vi "Read FTT Subpanel data.vi"(8 "error in (no error)":errorcluster, 11 "Main":T1={"Tite"="", "Base path"=path "", "Table"=[], "Stations"=[], "Shield Array"=[], "UPHs"=[], "VISA"={"VISA"="", "baud rate"=9600, "data bits"=8, "parity"=enum."None", "stop bits"=10, "flow control"=0}, "Path"={"roof"=path "", "Config"=path "", "Png"=path ""}, "Ctr"={"DB Dispaly"=refnum, "Error Table"=refnum, "Display"=refnum, "Login"=refnum, "Exit"=refnum, "FTT_Submit"=refnum}, "Login"={"User"="", "Grade"=""}, "information"={"cause"="", "Type"=enum."Inform", "code"=0, "Suroce"="", "Status"=FALSE}, "Local DB"={"Connstr"="", "Database"={"Constr"={"Driver"="", "Server"="", "User"="", "Pwd"="", "Database"=""}, "conn ref"=refnum, "State"=FALSE}}, "Remote DB"={"Connstr"="", "Database"={"Constr"={"Driver"="", "Server"="", "User"="", "Pwd"="", "Database"=""}, "conn ref"=refnum, "State"=FALSE}}, "FTT TV"="", "ExchangeTime"=0, "NVH"="", "EOL Path"=path ""} {"VISA"."flow control" items=["None", "XON/XOFF", "RTS/CTS", "XON/XOFF & RTS/CTS", "DTR/DSR", "XON/XOFF & DTR/DSR"]; "VISA"."stop bits" items=["1.0"=10, "1.5"=15, "2.0"=20]}) -> (0 "error out":errorcluster)   [LabVIEW 2014]
uses:
  Type'def/FTT Display Type.ctl
  <vilib>/addons/database/_DB Variant To Data/Database Variant To Data.xnode
  Type'def/UPH Config.ctl
  VISA/Ctr/VISA Ctr.ctl
  Type'def/Main Ctr Ref.ctl
  Type'def/User Login.ctl
  Database/Ctr/Constr.ctl
  <vilib>/addons/database/Connection.llb/Conn ObjectReference.ctl
  <vilib>/addons/database/NI_Database_API.lvlib
  Database/Ctr/Conneect State.ctl
  Type'def/MainCtr.ctl
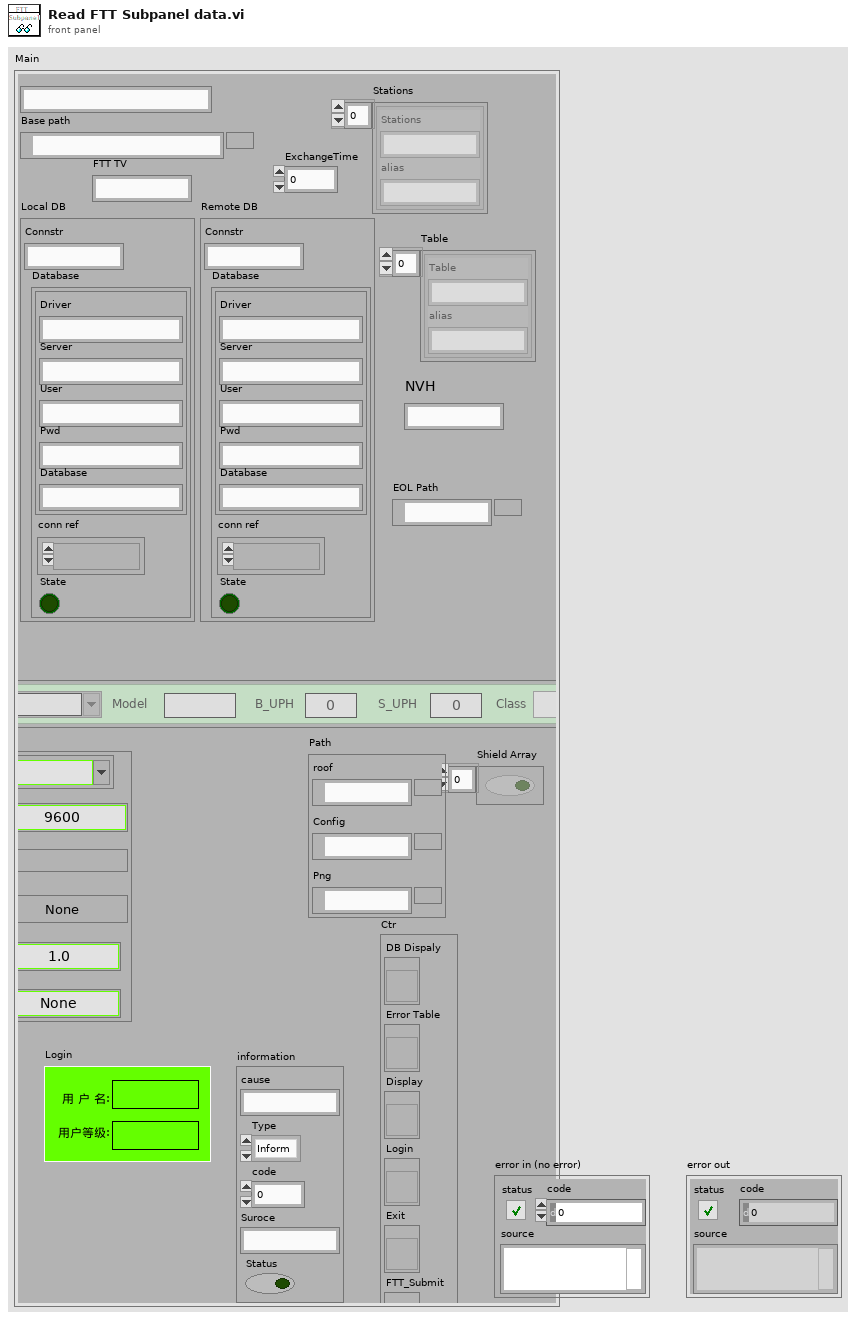
[diagram p1: front panel]
types:
  T1 = typedef "MainCtr.ctl" = cluster{"Tite":string, "Base path":path, "Table":cluster{"Table":string, "alias":string}[], "Stations":cluster{"Stations":string, "alias":string}[], "Shield Array":bool[], "UPHs":T2[], "VISA":T3, "Path":cluster{"roof":path, "Config":path, "Png":path}, "Ctr":T4, "Login":T5, "information":cluster{"cause":string, "Type":enum16{"Inform", "Warning", "Alarm"}, "code":i32, "Suroce":string, "Status":bool}, "Local DB":cluster{"Connstr":string, "Database":T6}, "Remote DB":cluster{"Connstr":string, "Database":T6}, "FTT TV":string, "ExchangeTime":i32, "NVH":string, "EOL Path":path}
  T2 = typedef "UPH Config.ctl" = cluster{"Line_No":string, "Model":string, "B_UPH ":i16, "S_UPH  ":i16, "Class":enum16{"Big", "Small"}}
  T3 = typedef "VISA Ctr.ctl" = cluster{"VISA":refnum<visa-resource-name>, "baud rate":u32, "data bits":u16, "parity":enum16{"None", "Odd", "Even", "Mark", "Space"}, "stop bits":u16, "flow control":u16}
  T4 = typedef "Main Ctr Ref.ctl" = cluster{"DB Dispaly":refnum<vi>, "Error Table":refnum<vi>, "Display":refnum<vi>, "Login":refnum<vi>, "Exit":refnum<vi>, "FTT_Submit":refnum<vi>}
  T5 = typedef "User Login.ctl" = cluster{"User":string, "Grade":string}
  T6 = typedef "Conneect State.ctl" = cluster{"Constr":T7, "conn ref":T8, "State":bool}
  T7 = typedef "Constr.ctl" = cluster{"Driver":string, "Server":string, "User":string, "Pwd":string, "Database":string}
  T8 = typedef "NI_Database_API.lvlib/Conn ObjectReference.ctl" = refnum<k1>
  T9 = typedef "FTT Display Type.ctl" = cluster{"Line.No":string, "Model":string, "Color":string, "UPH":dbl, "Plan":dbl, "Target Rate":dbl, "Target ":dbl, "Actual":dbl, "FTT":dbl, "FTT Rate":dbl, "Repaired":dbl, "Reject":dbl, "Ouline":dbl, "Line State":string}
  T10 = cluster{"cause":string, "Type":enum16{"Inform", "Warning", "Alarm"}, "code":i32, "Suroce":string, "Status":bool}
  T11 = cluster{"Main ":T1, "Display":T9, "information":cluster{"cause":string, "Type":enum16{"Inform", "Warning", "Alarm"}, "code":i32, "Suroce":string, "Status":bool}}
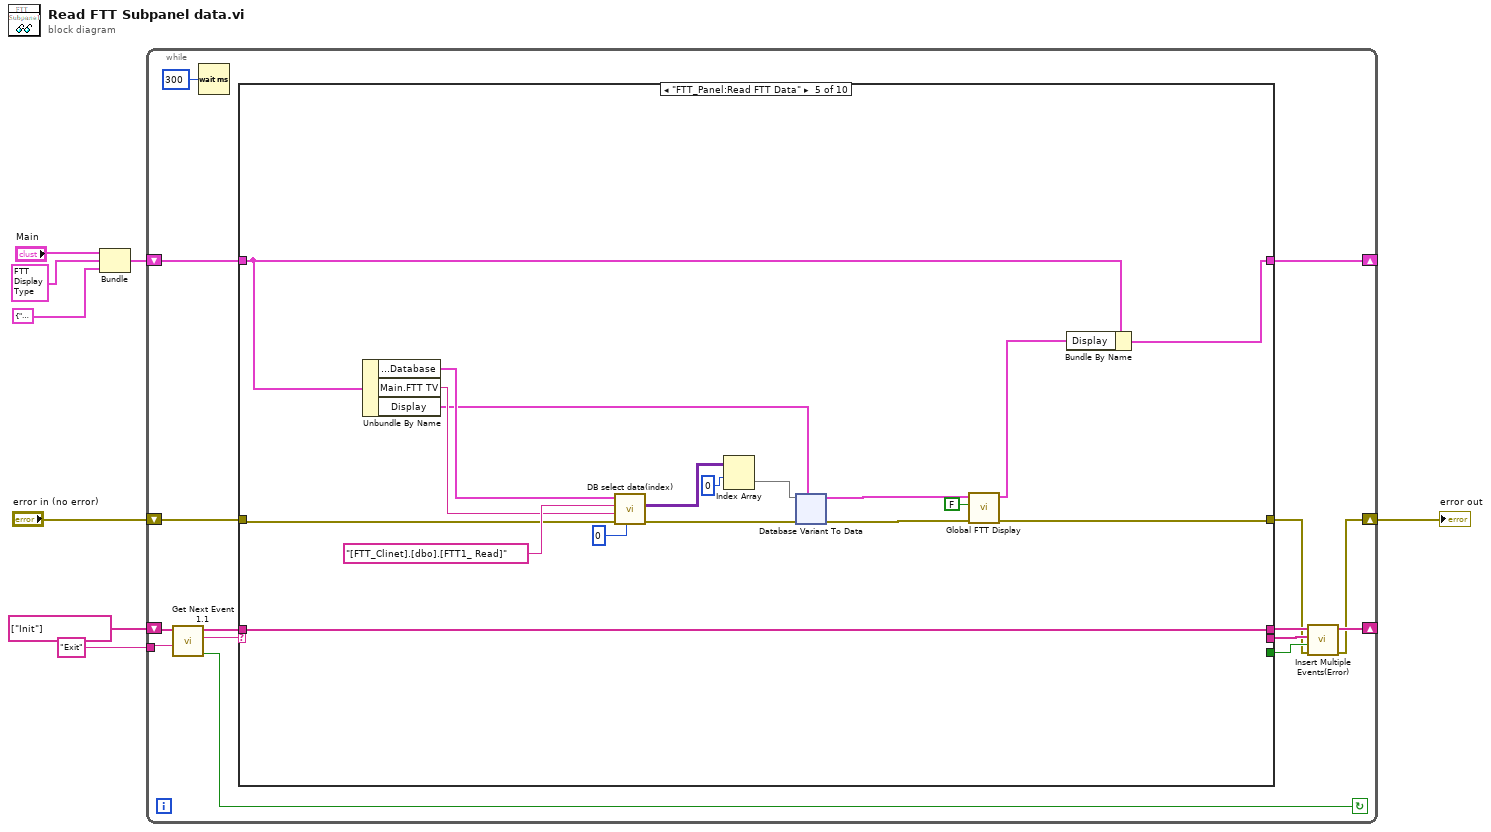
[diagram p0: block diagram]
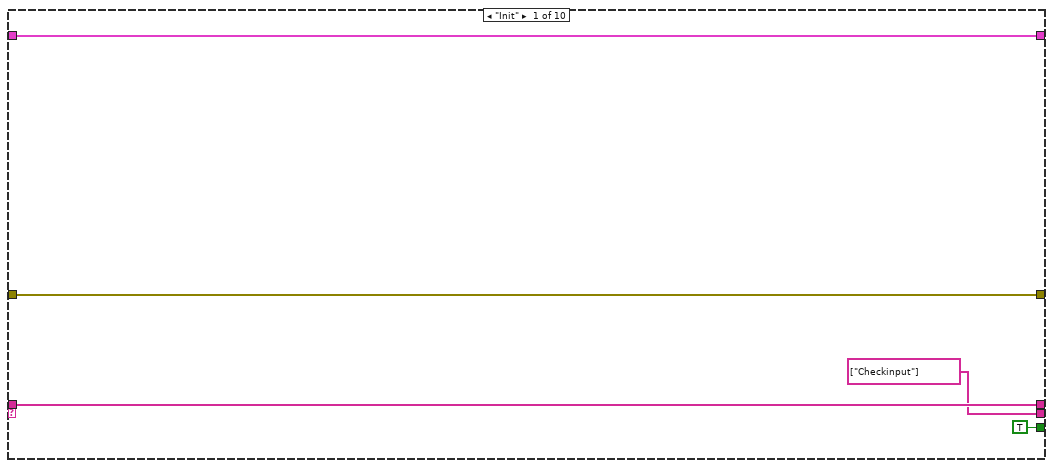
[diagram p2: hidden frame]
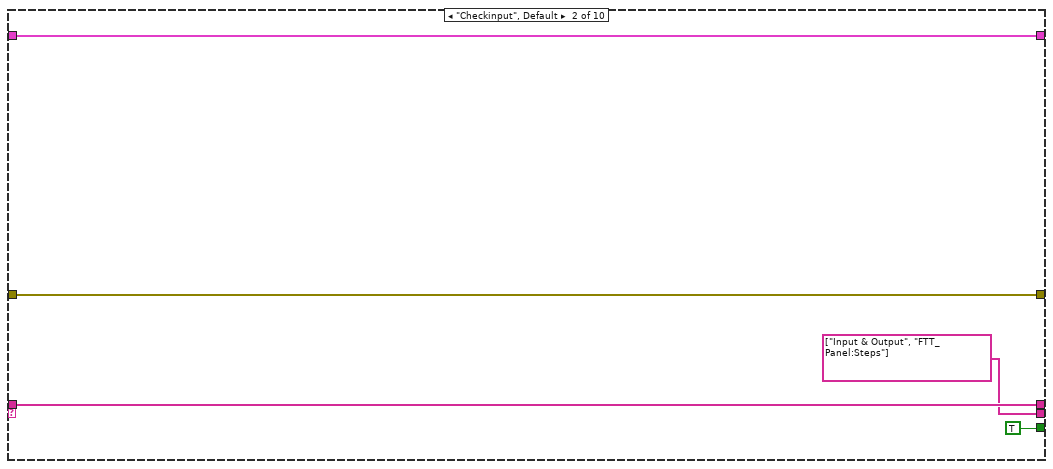
[diagram p3: hidden frame]
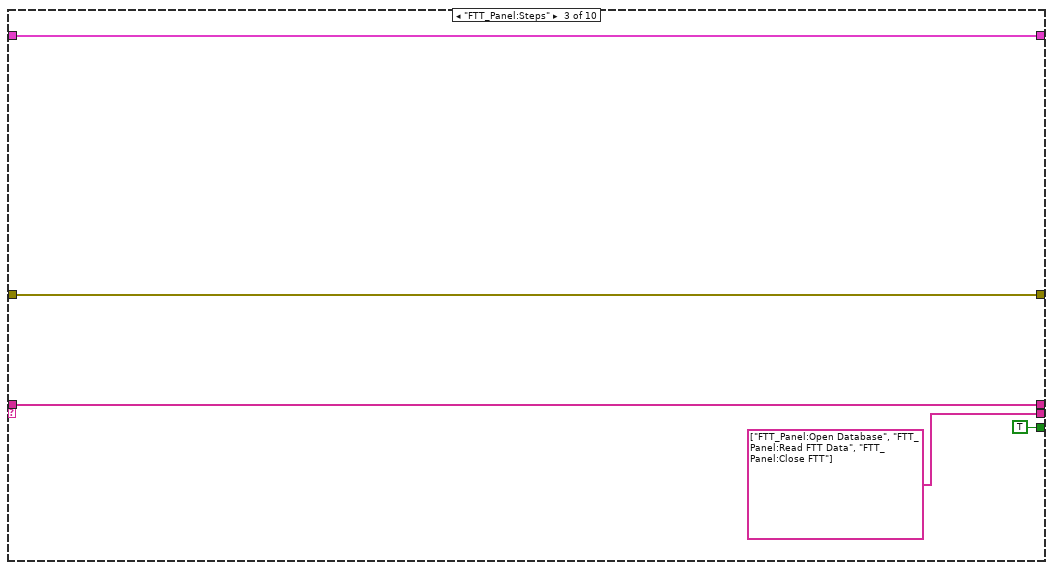
[diagram p4: hidden frame]
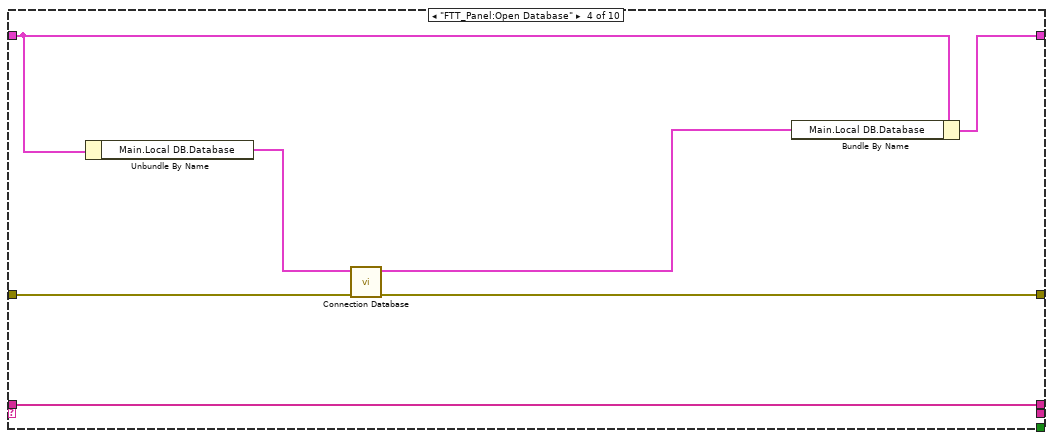
[diagram p5: hidden frame]
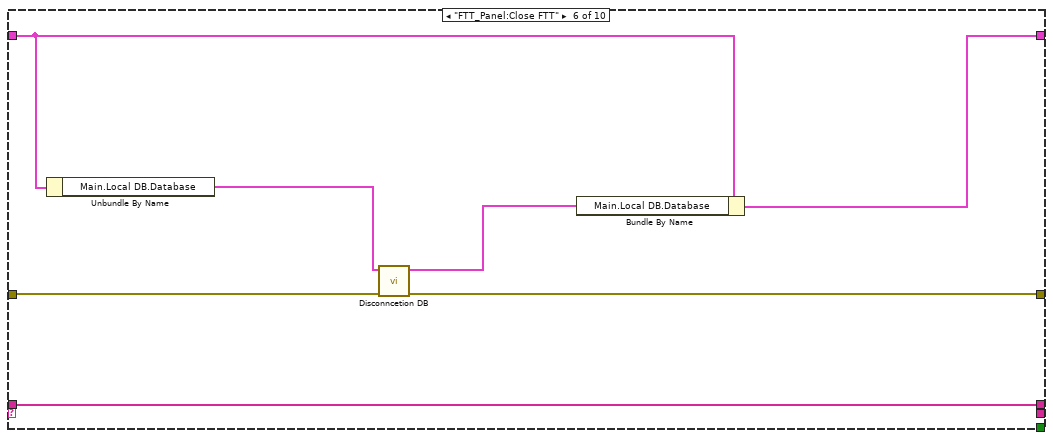
[diagram p6: hidden frame]
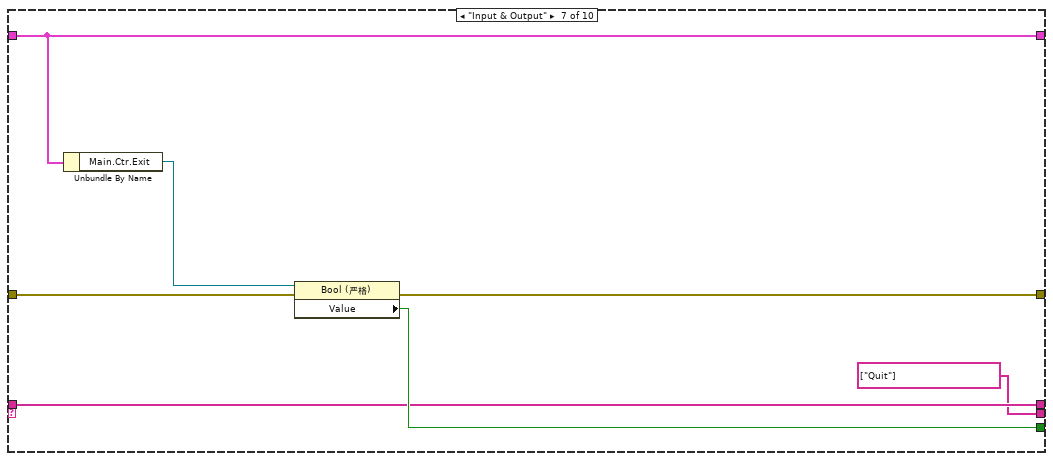
[diagram p7: hidden frame]
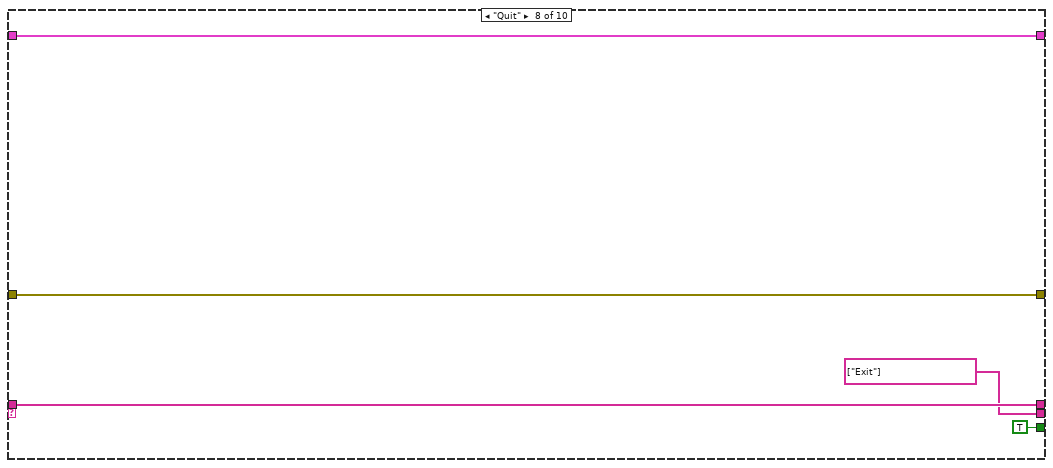
[diagram p8: hidden frame]
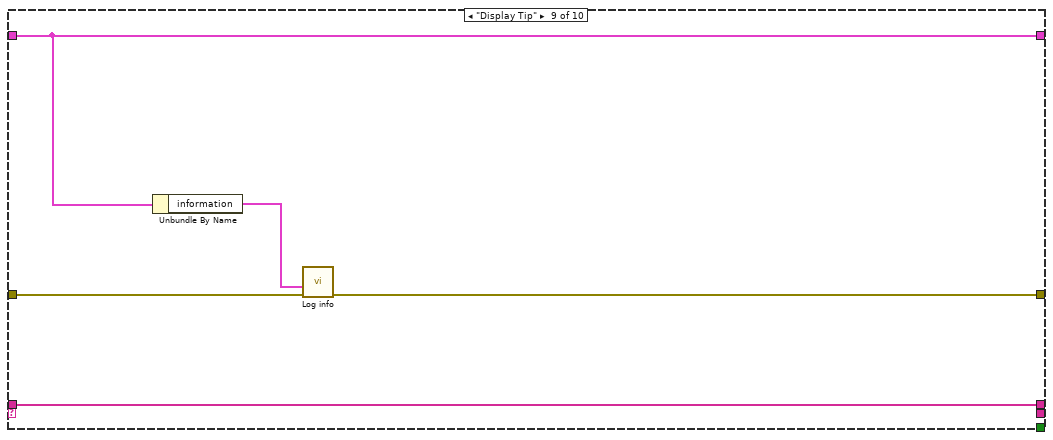
[diagram p9: hidden frame]
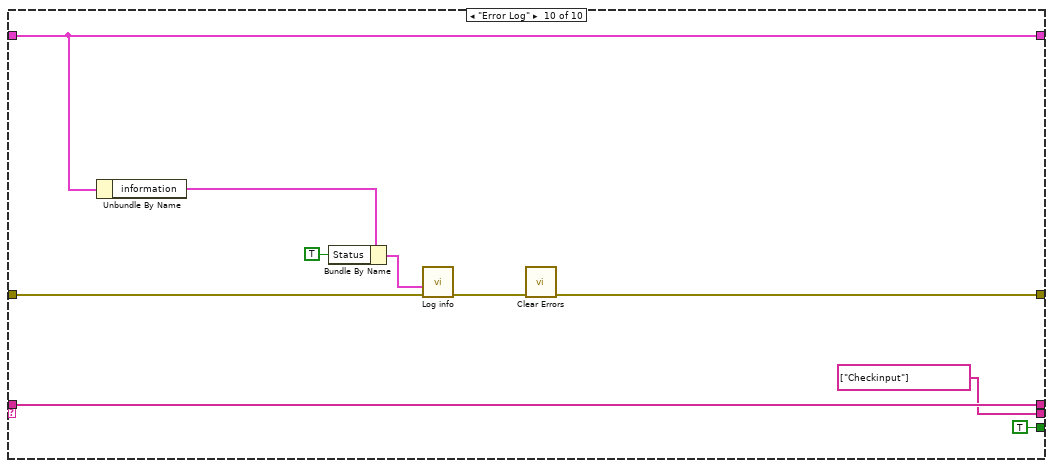
[diagram p10: hidden frame]
diagram:
  n1 = Bundle("Main"="Main", "Display"=T9 {"Line.No"="", "Model"="", "Color"="", "UPH"=0.0, "Plan"=0.0, "Target Rate"=0.0, "Target "=0.0, "Actual"=0.0, "FTT"=0.0, "FTT Rate"=0.0, "Repaired"=0.0, "Reject"=0.0, "Ouline"=0.0, "Line State"=""}, "information"=T10 {"cause"="", "Type"=enum."Inform", "code"=0, "Suroce"="", "Status"=FALSE}) -> (w5:T11)  [unwired: 1 in]
  n2 = while {
    tunnel: "Exit" ("Exit Event") -> [w20]
    shift-right: [w16] -> _
    shift-left: string[] ["Init"] -> [w21]
    shift-right: [w9] -> w3
    shift-left: "error in (no error)" -> [w19]
    shift-right: [w12] -> _
    shift-left: w5 -> [w17]
    stop <- w22 continue-if-true
    n3 = call "Get Next Event 1.1.vi"("Exit Event"=w20, "event queue in"=w21) -> ("Condition (Exit:F)"=w22:bool, "next event"=w23:string, "event queue out"=w18:string[])  [unwired: 6 in, 1 out]
    n4 = Wait (ms)(milliseconds to wait=u32 300) -> ()  [unwired: 1 out]
    n5 = case shown="\"FTT_Panel:Read FTT Data\"" w23 {
      tunnel: w19 -> [w26 w30 w37 w45 w58 w508 w514 w519 w525 w535]
      tunnel: w18 -> [w28 w33 w36 w42 w52 w505 w511 w518 w521 w528]
      tunnel: w17 -> [w27 w31 w38 w41 w54 w503 w515 w520 w523 w532]
      tunnel: [w26 w30 w37 w43 w50 w506 w510 w519 w524 w533] -> w10
      tunnel: [w28 w33 w36 w42 w52 w505 w511 w518 w521 w528] -> w15
      tunnel: [TRUE ("Insert all? (T)") TRUE ("Insert all? (T)") TRUE ("Insert all? (T)") _ _ _ w512 TRUE ("Insert all? (T)") _ TRUE ("Insert all? (T)")] -> w14
      tunnel: [string[] ["Checkinput"] string[] ["Input & Output", "FTT_Panel:Steps"] string[] ["FTT_Panel:Open Database", "FTT_Panel:Read FTT Data", "FTT_Panel:Close FTT"] _ _ _ string[] ["Quit"] string[] ["Exit"] _ string[] ["Checkinput"]] -> w13
      tunnel: [w27 w31 w38 w39 w53 w502 w515 w520 w523 w532] -> w12
      frame "Init" {
      }
      frame "Checkinput", Default {
      }
      frame "FTT_Panel:Steps" {
      }
      frame "FTT_Panel:Open Database" {
        n6 = Unbundle By Name(w41) -> ("Main.Local DB.Database"=w44:T6)
        n7 = call "Connection Database.vi"("error in (no error)"=w45, "Connncet State"=w44) -> ("error out"=w43:errorcluster, "Connncet State out"=w40:T6)  [unwired: 8 in]
        n8 = Bundle By Name(cluster=w41, "Main.Local DB.Database"=w40) -> (w39:T11)
      }
      frame "FTT_Panel:Read FTT Data" {
        n9 = Unbundle By Name(w54) -> ("Main.Local DB.Database"=w63:T6, "Main.FTT TV"=w61:string, "Display"=w55:T9)
        n10 = call "DB select data(index).vi"("index"=0, "error in (no error)"=w58, "Code"=w61, "Tabe"="[FTT_Clinet].[dbo].[FTT1_ Read]", "Connncet State"=w63) -> ("error out"=w57:errorcluster, "data"=w59:variant[][])  [unwired: 3 in, 2 out]
        n11 = Index Array(array=w59, index (row)=0 ("disabled index (col)")) -> (element=w56:variant[])  [unwired: 1 in]
        n12 = xnode "Database Variant To Data"("database variant"=w56, "error in (no error)"=w57, "type"=w55) -> ("data"=w49:T9, "error out"=w51:errorcluster)
        n13 = call "Global FTT Display.vi"("error in (no error)"=w51, "W/R"=FALSE, "Display"=w49) -> ("error out"=w50:errorcluster, "Display OUT"=w48:T9)  [unwired: 7 in]
        n14 = Bundle By Name(cluster=w54, "Display"=w48) -> (w53:T11)
      }
      frame "FTT_Panel:Close FTT" {
        n15 = Unbundle By Name(w503) -> ("Main.Local DB.Database"=w507:T6)
        n16 = call "Disconncetion DB.vi"("error in (no error)"=w508, "Connncet State"=w507) -> ("error out"=w506:errorcluster, "Connect State"=w504:T6)  [unwired: 8 in]
        n17 = Bundle By Name(cluster=w503, "Main.Local DB.Database"=w504) -> (w502:T11)
      }
      frame "Input & Output" {
        n18 = Unbundle By Name(w515) -> ("Main.Ctr.Exit"=w513:refnum<vi>)
        n19 = property class="Bool (严格)"(reference=w513, error in=w514) -> (error out=w510:errorcluster, "Value"=w512:bool)  [unwired: 1 out]
      }
      frame "Quit" {
      }
      frame "Display Tip" {
        n20 = Unbundle By Name(w523) -> ("information"=w522:T10)
        n21 = call "Log info.vi"("error in (no error)"=w525, "information"=w522) -> ("error out"=w524:errorcluster)  [unwired: 8 in, 1 out]
      }
      frame "Error Log" {
        n22 = Unbundle By Name(w532) -> ("information"=w531:T10)
        n23 = Bundle By Name(cluster=w531, "Status"=TRUE) -> (w530:T10)
        n24 = call "Log info.vi"("error in (no error)"=w535, "information"=w530) -> ("error out"=w534:errorcluster)  [unwired: 8 in, 1 out]
        n25 = call <vilib>:"Clear Errors.vi"("error in (no error)"=w534) -> ("error out"=w533:errorcluster)  [unwired: 5 in, 1 out]
      }
    }
    n26 = call "Insert Multiple Events(Error).vi"("error in (no error)"=w10, "Insert all? (T)"=w14, "Events to Insert"=w13, "Event queue in"=w15) -> ("error out"=w9:errorcluster, "Event queue out"=w16:string[])  [unwired: 6 in]
  }
  "error out" <- w3
